vi "Replace Population with Offspring.vi"(8 "error in (no error)":errorcluster, 11 "GA in":refnum<class "GA.lvclass">) -> (0 "error out":errorcluster, 3 "GA out":refnum<class "GA.lvclass">)   [LabVIEW 2013, in "GA.lvclass"]
uses:
  GA.lvclass
  GA.lvclass/GA.ctl
  Controls/Solution_GA.ctl
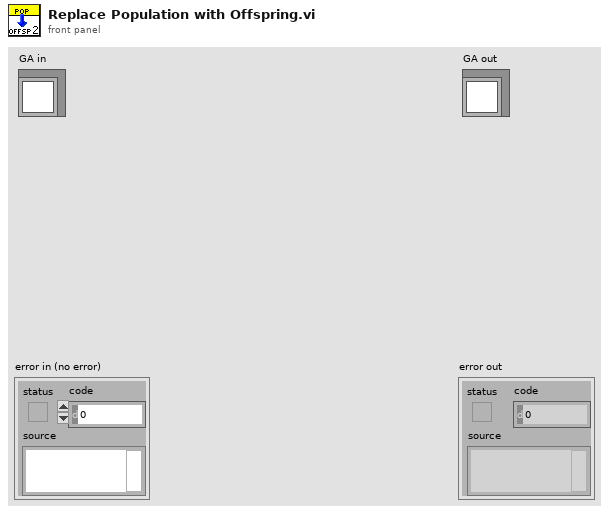
[diagram p1: front panel]
types:
  T1 = typedef "Solution_GA.ctl" = cluster{"Schedule":u16[], "Fitness":u16, "Fitness Valid?":bool}
  T2 = typedef "Strategy.ctl" = enum16{"Total Replacement", "Incremental Replacement", "Ellitist 1", "Elitist 2", "%10", "%20", "%30", "%40", "%50"}
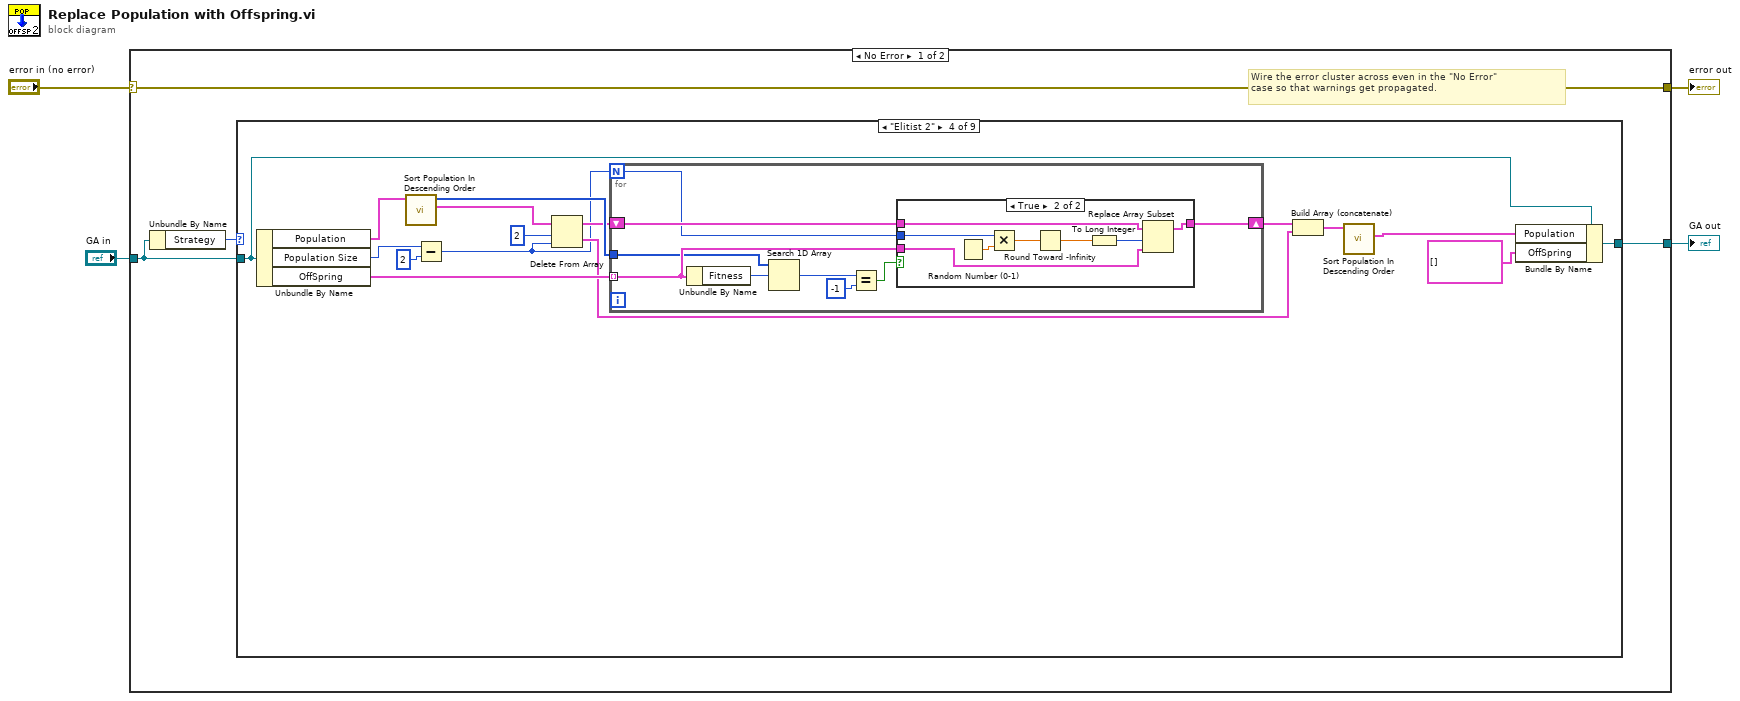
[diagram p0: block diagram]
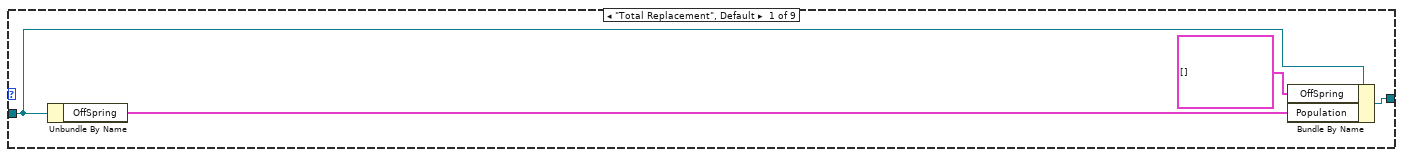
[diagram p2: hidden frame]
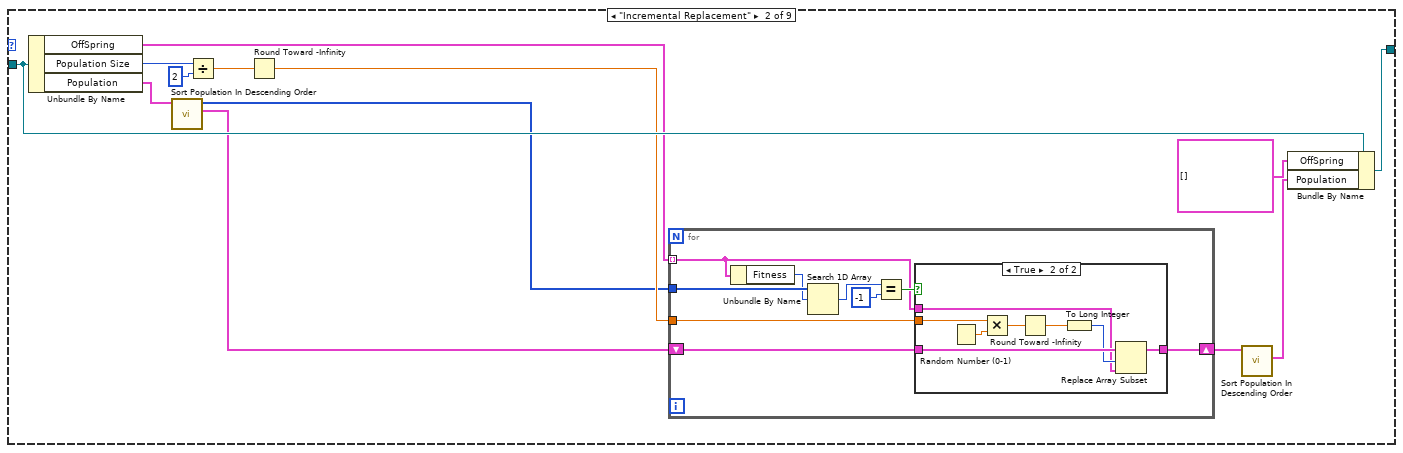
[diagram p3: hidden frame]
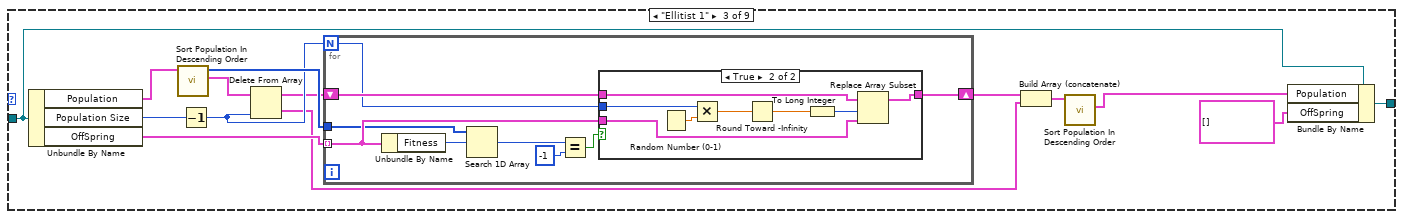
[diagram p5: hidden frame]
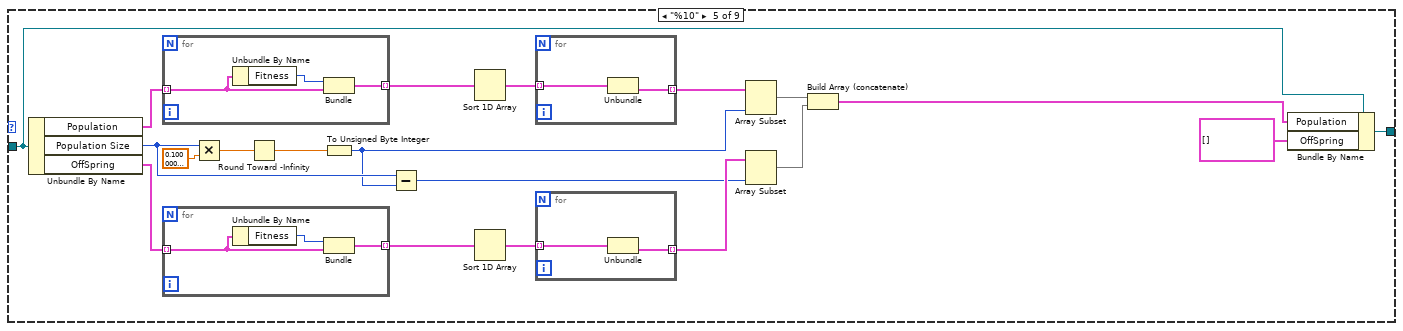
[diagram p8: hidden frame]
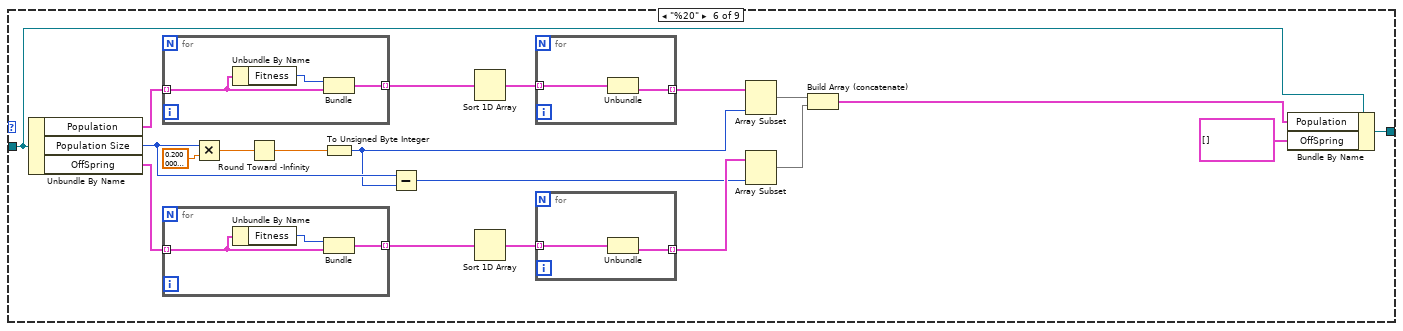
[diagram p9: hidden frame]
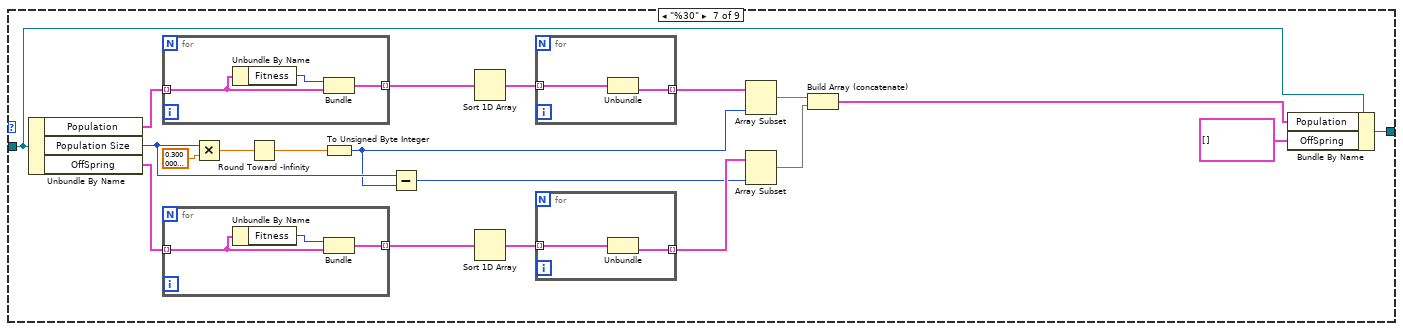
[diagram p10: hidden frame]
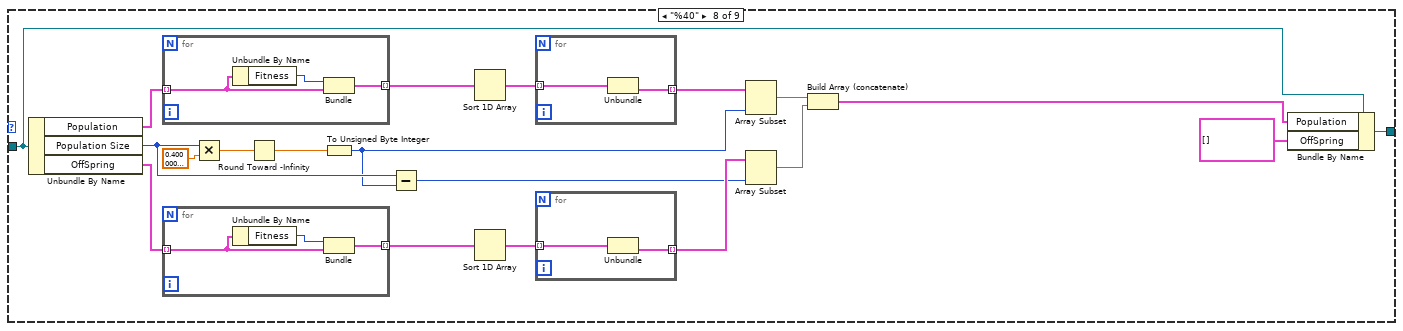
[diagram p11: hidden frame]
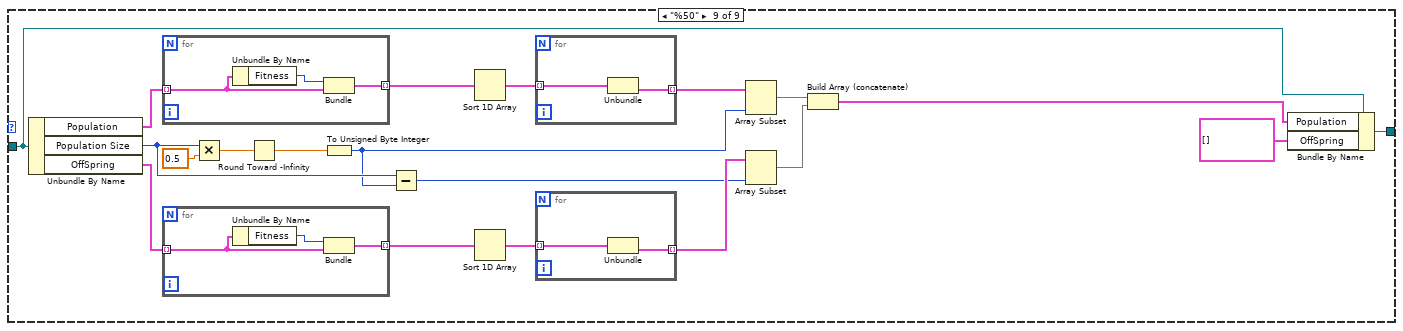
[diagram p12: hidden frame]
diagram:
  n1 = case shown="No Error" "error in (no error)" {
    selector: "error in (no error)" -> [w8 w261]
    tunnel: [w8 w261] -> w3
    tunnel: [w7 w260] -> w1
    tunnel: "GA in" -> [w6 w260]
    frame No Error {
      # "Wire the error cluster across even in the \"No Error\"\ncase so that warnings get propagated."
      n2 = Unbundle By Name(w6) -> ("Strategy"=w5:T2)
      n3 = case shown="\"Elitist 2\"" w5 {
        tunnel: w6 -> [w12 w25 w56 w91 w126 w156 w186 w216 w246]
        tunnel: [w11 w24 w55 w90 w125 w155 w185 w215 w245] -> w7
        frame "Total Replacement", Default {
          n4 = Unbundle By Name(w12) -> ("OffSpring"=w9:T1[])
          n5 = Bundle By Name(cluster=w12, "OffSpring"=T1[] [], "Population"=w9) -> (w11:refnum<class "GA.lvclass">)
        }
        frame "Incremental Replacement" {
          n6 = Unbundle By Name(w25) -> ("OffSpring"=w22:T1[], "Population Size"=w19:u8, "Population"=w17:T1[])
          n7 = call "Sort Population In Descending Order.vi"("Population"=w17) -> ("Population In Descending Order"=w15:T1[], "Fitness Values In Descending Order"=w16:u16[])  [unwired: 9 in]
          n8 = Divide(x=w19, y=u8 2) -> (x/y=w20:dbl)
          n9 = Round Toward -Infinity(1:w20) -> (0:w18:dbl)
          n10 = for {
            tunnel: w22 -> [w26] mode=indexing
            tunnel: w16 -> [w34]
            shift-right: [w32] -> w14
            shift-left: w15 -> [w33]
            tunnel: w18 -> [w27]
            n11 = Unbundle By Name(w26) -> ("Fitness"=w31:u16)
            n12 = Search 1D Array(1D array=w34, element=w31) -> (index of element=w30:i32)  [unwired: 1 in]
            n13 = Equal?(x=w30, y=-1) -> (x = y?=w28:bool)
            n14 = case shown="True" w28 {
              tunnel: w33 -> [w35 w42]
              tunnel: [w35 w43] -> w32
              tunnel: w27 -> [_ w39]
              tunnel: w26 -> [_ w36]
              frame False {
              }
              frame True {
                n15 = Random Number (0-1)() -> (number: 0 to 1=w40:dbl)
                n16 = Multiply(x=w39, y=w40) -> (x*y=w41:dbl)
                n17 = Round Toward -Infinity(1:w41) -> (0:w38:dbl)
                n18 = To Long Integer(number=w38) -> (32bit integer=w37:i32)
                n19 = Replace Array Subset(array=w42, new element=w36, index=w37) -> (w43:T1[])
              }
            }
          }
          n20 = call "Sort Population In Descending Order.vi"("Population"=w14) -> ("Population In Descending Order"=w13:T1[])  [unwired: 9 in, 1 out]
          n21 = Bundle By Name(cluster=w25, "OffSpring"=T1[] [], "Population"=w13) -> (w24:refnum<class "GA.lvclass">)
        }
        frame "Ellitist 1" {
          n22 = Unbundle By Name(w56) -> ("Population"=w53:T1[], "Population Size"=w57:u8, "OffSpring"=w52:T1[])
          n23 = call "Sort Population In Descending Order.vi"("Population"=w53) -> ("Population In Descending Order"=w50:T1[], "Fitness Values In Descending Order"=w51:u16[])  [unwired: 9 in]
          n24 = Decrement(x=w57) -> (x-1=w49:u8)
          n25 = Delete From Array(array=w50, index=w49) -> (deleted portion=w47:T1, array with subset deleted=w46:T1[])  [unwired: 1 in]
          n26 = for {
            N: w49 -> [w58]
            shift-right: [w65] -> w48
            shift-left: w46 -> [w66]
            tunnel: w52 -> [w60] mode=indexing
            tunnel: w51 -> [w59]
            n27 = Unbundle By Name(w60) -> ("Fitness"=w64:u16)
            n28 = Search 1D Array(1D array=w59, element=w64) -> (index of element=w63:i32)  [unwired: 1 in]
            n29 = Equal?(x=w63, y=-1) -> (x = y?=w61:bool)
            n30 = case shown="True" w61 {
              tunnel: w66 -> [w67 w69]
              tunnel: [w67 w75] -> w65
              tunnel: w60 -> [_ w70]
              tunnel: w58 -> [_ w68]
              frame False {
              }
              frame True {
                n31 = Random Number (0-1)() -> (number: 0 to 1=w73:dbl)
                n32 = Multiply(x=w68, y=w73) -> (x*y=w74:dbl)
                n33 = Round Toward -Infinity(1:w74) -> (0:w72:dbl)
                n34 = To Long Integer(number=w72) -> (32bit integer=w71:i32)
                n35 = Replace Array Subset(array=w69, new element=w70, index=w71) -> (w75:T1[])
              }
            }
          }
          n36 = Build Array (concatenate)(w48, w47) -> (w45:T1[])
          n37 = call "Sort Population In Descending Order.vi"("Population"=w45) -> ("Population In Descending Order"=w44:T1[])  [unwired: 9 in, 1 out]
          n38 = Bundle By Name(cluster=w56, "Population"=w44, "OffSpring"=T1[] []) -> (w55:refnum<class "GA.lvclass">)
        }
        frame "Elitist 2" {
          n39 = Unbundle By Name(w91) -> ("Population"=w88:T1[], "Population Size"=w79:u8, "OffSpring"=w87:T1[])
          n40 = call "Sort Population In Descending Order.vi"("Population"=w88) -> ("Population In Descending Order"=w81:T1[], "Fitness Values In Descending Order"=w86:u16[])  [unwired: 9 in]
          n41 = Subtract(x=w79, y=u8 2) -> (x-y=w77:u8)
          n42 = Delete From Array(array=w81, length=2, index=w77) -> (deleted portion=w80:T1[], array with subset deleted=w84:T1[])
          n43 = for {
            N: w77 -> [w92]
            shift-right: [w99] -> w85
            shift-left: w84 -> [w100]
            tunnel: w87 -> [w94] mode=indexing
            tunnel: w86 -> [w93]
            n44 = Unbundle By Name(w94) -> ("Fitness"=w98:u16)
            n45 = Search 1D Array(1D array=w93, element=w98) -> (index of element=w97:i32)  [unwired: 1 in]
            n46 = Equal?(x=w97, y=-1) -> (x = y?=w95:bool)
            n47 = case shown="True" w95 {
              tunnel: w100 -> [w101 w103]
              tunnel: [w101 w109] -> w99
              tunnel: w94 -> [_ w104]
              tunnel: w92 -> [_ w102]
              frame False {
              }
              frame True {
                n48 = Random Number (0-1)() -> (number: 0 to 1=w107:dbl)
                n49 = Multiply(x=w102, y=w107) -> (x*y=w108:dbl)
                n50 = Round Toward -Infinity(1:w108) -> (0:w106:dbl)
                n51 = To Long Integer(number=w106) -> (32bit integer=w105:i32)
                n52 = Replace Array Subset(array=w103, new element=w104, index=w105) -> (w109:T1[])
              }
            }
          }
          n53 = Build Array (concatenate)(w85, w80) -> (w83:T1[])
          n54 = call "Sort Population In Descending Order.vi"("Population"=w83) -> ("Population In Descending Order"=w82:T1[])  [unwired: 9 in, 1 out]
          n55 = Bundle By Name(cluster=w91, "Population"=w82, "OffSpring"=T1[] []) -> (w90:refnum<class "GA.lvclass">)
        }
        frame "%10" {
          n56 = Unbundle By Name(w126) -> ("Population"=w129:T1[], "Population Size"=w116:u8, "OffSpring"=w123:T1[])
          n57 = for {
            tunnel: w129 -> [w138] mode=indexing
            tunnel: [w137] -> w128 mode=indexing
            n58 = Unbundle By Name(w138) -> ("Fitness"=w139:u16)
            n59 = Bundle("Fitness"=w139, "Solution"=w138) -> (w137:cluster{"Fitness":u16, "Solution":T1})  [unwired: 1 in]
          }
          n60 = for {
            tunnel: w123 -> [w133] mode=indexing
            tunnel: [w132] -> w122 mode=indexing
            n61 = Unbundle By Name(w133) -> ("Fitness"=w134:u16)
            n62 = Bundle("Fitness"=w134, "Solution"=w133) -> (w132:cluster{"Fitness":u16, "Solution":T1})  [unwired: 1 in]
          }
          n63 = Multiply(x=w116, y=sgl 0.1) -> (x*y=w119:sgl)
          n64 = Round Toward -Infinity(1:w119) -> (0:w118:sgl)
          n65 = To Unsigned Byte Integer(number=w118) -> (unsigned 8bit integer=w115:u8)
          n66 = Subtract(x=w116, y=w115) -> (x-y=w113:u8)
          n67 = Sort 1D Array(array=w128) -> (sorted array=w127:cluster{"Fitness":u16, "Solution":T1}[])
          n68 = Sort 1D Array(array=w122) -> (sorted array=w121:cluster{"Fitness":u16, "Solution":T1}[])
          n69 = for {
            tunnel: w127 -> [w136] mode=indexing
            tunnel: [w135] -> w117 mode=indexing
            n70 = Unbundle(w136) -> ("Solution"=w135:T1)  [unwired: 1 out]
          }
          n71 = for {
            tunnel: w121 -> [w131] mode=indexing
            tunnel: [w130] -> w114 mode=indexing
            n72 = Unbundle(w131) -> ("Solution"=w130:T1)  [unwired: 1 out]
          }
          n73 = Array Subset(array=w117, length=w115) -> (w112:T1[])  [unwired: 1 in]
          n74 = Array Subset(array=w114, length=w113) -> (w111:T1[])  [unwired: 1 in]
          n75 = Build Array (concatenate)(w112, w111) -> (w110:T1[])
          n76 = Bundle By Name(cluster=w126, "Population"=w110, "OffSpring"=T1[] []) -> (w125:refnum<class "GA.lvclass">)
        }
        frame "%20" {
          n77 = Unbundle By Name(w156) -> ("Population"=w159:T1[], "Population Size"=w146:u8, "OffSpring"=w153:T1[])
          n78 = for {
            tunnel: w159 -> [w168] mode=indexing
            tunnel: [w167] -> w158 mode=indexing
            n79 = Unbundle By Name(w168) -> ("Fitness"=w169:u16)
            n80 = Bundle("Fitness"=w169, "Solution"=w168) -> (w167:cluster{"Fitness":u16, "Solution":T1})  [unwired: 1 in]
          }
          n81 = for {
            tunnel: w153 -> [w163] mode=indexing
            tunnel: [w162] -> w152 mode=indexing
            n82 = Unbundle By Name(w163) -> ("Fitness"=w164:u16)
            n83 = Bundle("Fitness"=w164, "Solution"=w163) -> (w162:cluster{"Fitness":u16, "Solution":T1})  [unwired: 1 in]
          }
          n84 = Multiply(x=w146, y=sgl 0.2) -> (x*y=w149:sgl)
          n85 = Round Toward -Infinity(1:w149) -> (0:w148:sgl)
          n86 = To Unsigned Byte Integer(number=w148) -> (unsigned 8bit integer=w145:u8)
          n87 = Subtract(x=w146, y=w145) -> (x-y=w143:u8)
          n88 = Sort 1D Array(array=w158) -> (sorted array=w157:cluster{"Fitness":u16, "Solution":T1}[])
          n89 = Sort 1D Array(array=w152) -> (sorted array=w151:cluster{"Fitness":u16, "Solution":T1}[])
          n90 = for {
            tunnel: w157 -> [w166] mode=indexing
            tunnel: [w165] -> w147 mode=indexing
            n91 = Unbundle(w166) -> ("Solution"=w165:T1)  [unwired: 1 out]
          }
          n92 = for {
            tunnel: w151 -> [w161] mode=indexing
            tunnel: [w160] -> w144 mode=indexing
            n93 = Unbundle(w161) -> ("Solution"=w160:T1)  [unwired: 1 out]
          }
          n94 = Array Subset(array=w147, length=w145) -> (w142:T1[])  [unwired: 1 in]
          n95 = Array Subset(array=w144, length=w143) -> (w141:T1[])  [unwired: 1 in]
          n96 = Build Array (concatenate)(w142, w141) -> (w140:T1[])
          n97 = Bundle By Name(cluster=w156, "Population"=w140, "OffSpring"=T1[] []) -> (w155:refnum<class "GA.lvclass">)
        }
        frame "%30" {
          n98 = Unbundle By Name(w186) -> ("Population"=w189:T1[], "Population Size"=w176:u8, "OffSpring"=w183:T1[])
          n99 = for {
            tunnel: w189 -> [w198] mode=indexing
            tunnel: [w197] -> w188 mode=indexing
            n100 = Unbundle By Name(w198) -> ("Fitness"=w199:u16)
            n101 = Bundle("Fitness"=w199, "Solution"=w198) -> (w197:cluster{"Fitness":u16, "Solution":T1})  [unwired: 1 in]
          }
          n102 = for {
            tunnel: w183 -> [w193] mode=indexing
            tunnel: [w192] -> w182 mode=indexing
            n103 = Unbundle By Name(w193) -> ("Fitness"=w194:u16)
            n104 = Bundle("Fitness"=w194, "Solution"=w193) -> (w192:cluster{"Fitness":u16, "Solution":T1})  [unwired: 1 in]
          }
          n105 = Multiply(x=w176, y=sgl 0.3) -> (x*y=w179:sgl)
          n106 = Round Toward -Infinity(1:w179) -> (0:w178:sgl)
          n107 = To Unsigned Byte Integer(number=w178) -> (unsigned 8bit integer=w175:u8)
          n108 = Subtract(x=w176, y=w175) -> (x-y=w173:u8)
          n109 = Sort 1D Array(array=w188) -> (sorted array=w187:cluster{"Fitness":u16, "Solution":T1}[])
          n110 = Sort 1D Array(array=w182) -> (sorted array=w181:cluster{"Fitness":u16, "Solution":T1}[])
          n111 = for {
            tunnel: w187 -> [w196] mode=indexing
            tunnel: [w195] -> w177 mode=indexing
            n112 = Unbundle(w196) -> ("Solution"=w195:T1)  [unwired: 1 out]
          }
          n113 = for {
            tunnel: w181 -> [w191] mode=indexing
            tunnel: [w190] -> w174 mode=indexing
            n114 = Unbundle(w191) -> ("Solution"=w190:T1)  [unwired: 1 out]
          }
          n115 = Array Subset(array=w177, length=w175) -> (w172:T1[])  [unwired: 1 in]
          n116 = Array Subset(array=w174, length=w173) -> (w171:T1[])  [unwired: 1 in]
          n117 = Build Array (concatenate)(w172, w171) -> (w170:T1[])
          n118 = Bundle By Name(cluster=w186, "Population"=w170, "OffSpring"=T1[] []) -> (w185:refnum<class "GA.lvclass">)
        }
        frame "%40" {
          n119 = Unbundle By Name(w216) -> ("Population"=w219:T1[], "Population Size"=w206:u8, "OffSpring"=w213:T1[])
          n120 = for {
            tunnel: w219 -> [w228] mode=indexing
            tunnel: [w227] -> w218 mode=indexing
            n121 = Unbundle By Name(w228) -> ("Fitness"=w229:u16)
            n122 = Bundle("Fitness"=w229, "Solution"=w228) -> (w227:cluster{"Fitness":u16, "Solution":T1})  [unwired: 1 in]
          }
          n123 = for {
            tunnel: w213 -> [w223] mode=indexing
            tunnel: [w222] -> w212 mode=indexing
            n124 = Unbundle By Name(w223) -> ("Fitness"=w224:u16)
            n125 = Bundle("Fitness"=w224, "Solution"=w223) -> (w222:cluster{"Fitness":u16, "Solution":T1})  [unwired: 1 in]
          }
          n126 = Multiply(x=w206, y=sgl 0.4) -> (x*y=w209:sgl)
          n127 = Round Toward -Infinity(1:w209) -> (0:w208:sgl)
          n128 = To Unsigned Byte Integer(number=w208) -> (unsigned 8bit integer=w205:u8)
          n129 = Subtract(x=w206, y=w205) -> (x-y=w203:u8)
          n130 = Sort 1D Array(array=w218) -> (sorted array=w217:cluster{"Fitness":u16, "Solution":T1}[])
          n131 = Sort 1D Array(array=w212) -> (sorted array=w211:cluster{"Fitness":u16, "Solution":T1}[])
          n132 = for {
            tunnel: w217 -> [w226] mode=indexing
            tunnel: [w225] -> w207 mode=indexing
            n133 = Unbundle(w226) -> ("Solution"=w225:T1)  [unwired: 1 out]
          }
          n134 = for {
            tunnel: w211 -> [w221] mode=indexing
            tunnel: [w220] -> w204 mode=indexing
            n135 = Unbundle(w221) -> ("Solution"=w220:T1)  [unwired: 1 out]
          }
          n136 = Array Subset(array=w207, length=w205) -> (w202:T1[])  [unwired: 1 in]
          n137 = Array Subset(array=w204, length=w203) -> (w201:T1[])  [unwired: 1 in]
          n138 = Build Array (concatenate)(w202, w201) -> (w200:T1[])
          n139 = Bundle By Name(cluster=w216, "Population"=w200, "OffSpring"=T1[] []) -> (w215:refnum<class "GA.lvclass">)
        }
        frame "%50" {
          n140 = Unbundle By Name(w246) -> ("Population"=w249:T1[], "Population Size"=w236:u8, "OffSpring"=w243:T1[])
          n141 = for {
            tunnel: w249 -> [w258] mode=indexing
            tunnel: [w257] -> w248 mode=indexing
            n142 = Unbundle By Name(w258) -> ("Fitness"=w259:u16)
            n143 = Bundle("Fitness"=w259, "Solution"=w258) -> (w257:cluster{"Fitness":u16, "Solution":T1})  [unwired: 1 in]
          }
          n144 = for {
            tunnel: w243 -> [w253] mode=indexing
            tunnel: [w252] -> w242 mode=indexing
            n145 = Unbundle By Name(w253) -> ("Fitness"=w254:u16)
            n146 = Bundle("Fitness"=w254, "Solution"=w253) -> (w252:cluster{"Fitness":u16, "Solution":T1})  [unwired: 1 in]
          }
          n147 = Multiply(x=w236, y=sgl 0.5) -> (x*y=w239:sgl)
          n148 = Round Toward -Infinity(1:w239) -> (0:w238:sgl)
          n149 = To Unsigned Byte Integer(number=w238) -> (unsigned 8bit integer=w235:u8)
          n150 = Subtract(x=w236, y=w235) -> (x-y=w233:u8)
          n151 = Sort 1D Array(array=w248) -> (sorted array=w247:cluster{"Fitness":u16, "Solution":T1}[])
          n152 = Sort 1D Array(array=w242) -> (sorted array=w241:cluster{"Fitness":u16, "Solution":T1}[])
          n153 = for {
            tunnel: w247 -> [w256] mode=indexing
            tunnel: [w255] -> w237 mode=indexing
            n154 = Unbundle(w256) -> ("Solution"=w255:T1)  [unwired: 1 out]
          }
          n155 = for {
            tunnel: w241 -> [w251] mode=indexing
            tunnel: [w250] -> w234 mode=indexing
            n156 = Unbundle(w251) -> ("Solution"=w250:T1)  [unwired: 1 out]
          }
          n157 = Array Subset(array=w237, length=w235) -> (w232:T1[])  [unwired: 1 in]
          n158 = Array Subset(array=w234, length=w233) -> (w231:T1[])  [unwired: 1 in]
          n159 = Build Array (concatenate)(w232, w231) -> (w230:T1[])
          n160 = Bundle By Name(cluster=w246, "Population"=w230, "OffSpring"=T1[] []) -> (w245:refnum<class "GA.lvclass">)
        }
      }
    }
    frame Error {
    }
  }
  "error out" <- w3
  "GA out" <- w1
